vi "execution class name.vi"(8 "error in":errorcluster, 11 "System Diagnostics configuration in":refnum<class "System Diagnostics configuration.lvclass">) -> (0 "error out":errorcluster, 2 "class name":string, 3 "System Diagnostics configuration out":refnum<class "System Diagnostics configuration.lvclass">)   [LabVIEW 2013, in "System Diagnostics configuration.lvclass"]
doc: "Provides an interface for determining the module runtime class associated with this module configuration. This class name can then be used to dynamically load or locate the runtime class for initialization purposes."
uses:
  System Diagnostics configuration.lvclass
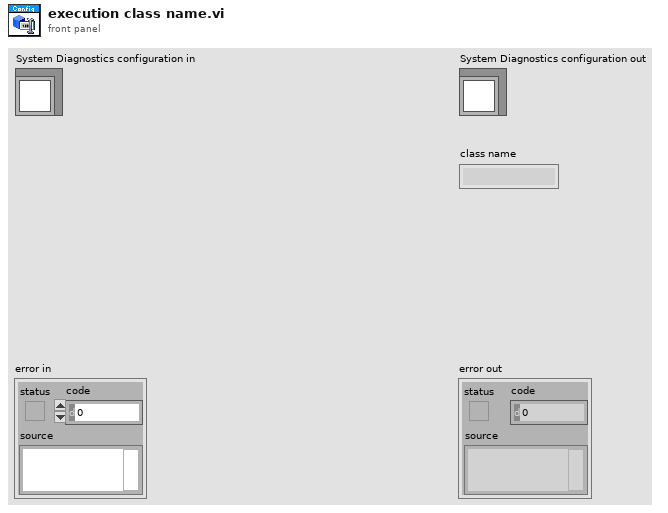
[diagram p1: front panel]
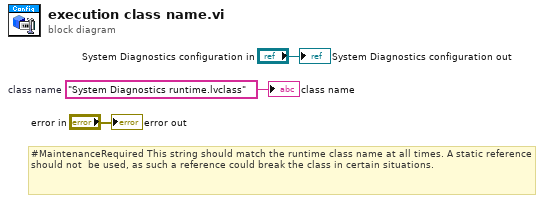
[diagram p0: block diagram]
diagram:
  w1 = "System Diagnostics runtime.lvclass"  # class name
  # "#MaintenanceRequired This string should match the runtime class name at all times. A static reference should not  be used, as such a reference could break the class in certain situations."
  "error out" <- "error in"
  "System Diagnostics configuration out" <- "System Diagnostics configuration in"
  "class name" <- w1
